vi "Process Thrust.vi"(11 "Arilou in":refnum<class "Slylandro.lvclass">) -> (3 "Arilou out":refnum<class "Slylandro.lvclass">)   [LabVIEW 2021, in "Slylandro.lvclass"]
uses:
  Slylandro.lvclass
  C:/dev/LabVIEW/LabMelee/Source/Application Specific/Element/Element.lvclass
  Element/Element.lvclass/Element.ctl
  Motion/Motion.lvclass/Motion.ctl
  Vector 2D/Vector 2D.lvclass/Vector 2D.ctl
  Element/Element.lvclass
  Motion/Motion.lvclass
  Vector 2D/Vector 2D.lvclass
panel:
  out "x+1":dbl
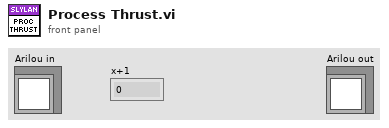
[diagram p1: front panel]
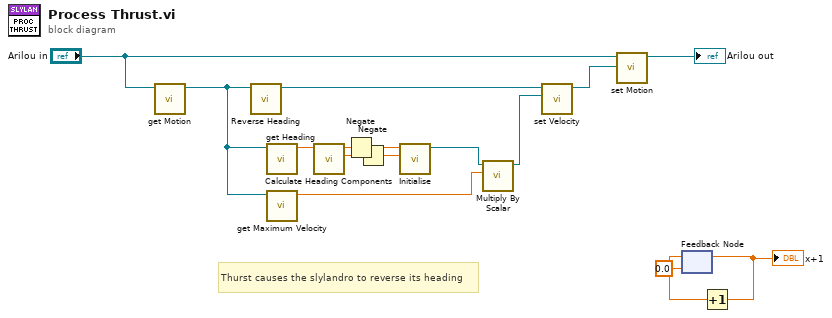
[diagram p0: block diagram]
diagram:
  # "Thurst causes the slylandro to reverse its heading"
  n1 = call "get Motion.vi"("Element in"="Arilou in") -> ("Motion"=w7:refnum<class "Motion.lvclass">)  [unwired: 10 in]
  n2 = call "Reverse Heading.vi"("Motion in"=w7) -> ("Motion out"=w10:refnum<class "Motion.lvclass">)  [unwired: 10 in]
  n3 = call "get Heading.vi"("Motion in"=w7) -> ("Heading [deg]"=w14:sgl)  [unwired: 10 in]
  n4 = call "get Maximum Velocity.vi"("Motion in"=w7) -> ("Maximum Velocity"=w6:sgl)  [unwired: 10 in]
  n5 = call "Calculate Heading Components.vi"("Heading In [deg]"=w14) -> ("Sin Heading"=w11:sgl, "Cos Heading"=w12:sgl)  [unwired: 9 in]
  n6 = Negate(x=w12) -> (-x=w9:sgl)
  n7 = Negate(x=w11) -> (-x=w8:sgl)
  n8 = call "Initialise.vi"("y"=w8, "x"=w9) -> ("Vector 2D out"=w5:refnum<class "Vector 2D.lvclass">)  [unwired: 9 in]
  n9 = call "Multiply By Scalar.vi"("x"=w6, "A"=w5) -> ("Ax"=w4:refnum<class "Vector 2D.lvclass">)  [unwired: 9 in]
  n10 = call "set Velocity.vi"("Velocity"=w4, "Motion in"=w10) -> ("Motion out"=w13:refnum<class "Motion.lvclass">)  [unwired: 9 in]
  n11 = call "set Motion.vi"("Motion"=w13, "Element in"="Arilou in") -> ("Element out"=→"Arilou out":refnum<class "Slylandro.lvclass">)  [unwired: 9 in]
  n12 = feedback #1(0.0) -> (w2:dbl)
  n13 = Increment(x=w2) -> (x+1=w3:dbl)
  "x+1" <- w3
  n14 = feedback-in #1(w3) -> ()
